vi "Eye Movement Analyser.vi"(7 "Data Output":T12) -> ()   [LabVIEW 2016] (continued)
              frame #1 {
                n995 = local read "Fixed Amplitude"() -> (w2031:bool)
                n996 = case shown="False" w2031 {
                  tunnel: [u8 0 ("Y Scale.Scale Fit") u8 2 ("Y Scale.Scale Fit")] -> w2032
                  frame True {
                  }
                  frame False {
                  }
                }
                n997 = property on="Impulse Trace" class="WFGraph (strict)"("Y Scale.Scale Fit"=w2032) -> ()  [unwired: 2 in, 2 out]
              }
              frame #2 {
                n998 = for {
                  tunnel: w2035 -> [w2041] mode=indexing
                  i -> [w2040]
                  w2036 = 3  # M-STD, M, M+STD
                  n999 = Unbundle By Name(w2041) -> ("Color"=w2038:u32, "Visible"=w2037:bool)
                  n1000 = Multiply(x=w2036, y=w2040) -> (x*y=w2039:i32)
                  n1001 = for {
                    N: w2036 -> [_]
                    tunnel: w2039 -> [w2049]
                    tunnel: w2038 -> [w2042]
                    tunnel: w2037 -> [w2048]
                    i -> [w2046]
                    n1002 = Add(x=w2046, y=w2049) -> (x+y=w2044:i32)
                    n1003 = Equal?(x=w2046, y=1) -> (x = y?=w2047:bool)
                    n1004 = case shown="True" w2047 {
                      tunnel: [u8 0 ("Plot.Line Width") u8 5 ("Plot.Line Width")] -> w2043
                      frame False {
                      }
                      frame True {
                      }
                    }
                    n1005 = property on="Impulse Trace" class="WFGraph (strict)"("Active Plot"=w2044, "Plot.Plot Color"=w2042, "Plot.Visible"=w2048, "Plot.Line Width"=w2043, "Plot.Fill/Pt. Color"=w2042) -> ()  [unwired: 2 in, 2 out]
                  }
                }
              }
            }
          }
          frame Enabled {
          }
        }
      }
      frame "Gain and Phase" {
        n1006 = Bundle By Name(cluster=w2055, "Session saved?"=FALSE) -> (w2054:T17)
        n1007 = local read "Trace"() -> (w2059:i32)
        n1008 = call "Data Analysis.vi"("Data IN"=w2058, "Trace Select"=w2059) -> ("Data OUT"=w2057:T30)  [unwired: 13 in]
      }
      frame "Time Constant Plugin" {
        n1009 = call "Ema to Plugin Data Converter.vi"("Data OUT"=w2064) -> ("Shared Data from EMA"=w2066:T47)  [unwired: 10 in]
        n1010 = Bundle By Name(cluster=w2068, "Session saved?"=FALSE) -> (w2062:T17)
        n1011 = disable-structure shown="Enabled" {
          disable-tunnel: w2066 -> [w2072 w2073]
          disable-tunnel: [w2071 w2073] -> w2065
          frame Disabled {
            n1012 = call "Time Constant - Plugin Main.vi"("Shared Data from EMA"=w2072) -> ("Shared Data to EMA"=w2071:T48)  [unwired: 10 in]
          }
          frame Enabled {
          }
        }
        n1013 = call "Plugin to Ema Data Converter.vi"("Shared Data from EMA in"=w2065, "Data OUT in"=w2064) -> ("Data OUT out"=w2063:T30)  [unwired: 9 in]
      }
      frame "Desaccade Time Data" {
        w2074 = T14[] [enum."Generate New Time Plot", enum."Generate New Impulse Plot"] items=["--- System ---", "Panel Monitoring", "Check Save Status", "Initialize", "Initialise GUI", "Quit", "--- Import ---", "Desaccade Time Data", "Desaccade Time Data Background", "Paint Delete", "Load Batch Log File", "Make Batch List", "Update Batch List", "Delete Batch List", "Delete Temporary LVS", "Save Temporary LVS", "Check for Batch LVS", "Process 3D Chinchilla", "Find default parameter", "Mars3D old", "Chair", "EyeSeeCam", "Open last session", "Save RAW", "Auto Impulse Parameter", "Save Image", "Wireless", "Process Coils Data", "Process JHOC Data", "Process Animal Data", "Australian Data", "ASCII", "Mars 3D", "Mars 3D Training", "Position Mean Plugin", "plot generator plugin", "Human VOG system", "Optotrak", "spline", "COR", "galvanic", "Generate New Time Plot", "Make off and gains permanent", "Generate New Impulse Plot", "Defer Impulse Plot", "Fill Impulse Plot Data", "Scale Impulse Plot", "Un-Defer Impulse Plot", "Snap Impulse Cursor", "Extract Saccades", "Impulse Analyser", "NTA", "Acceleration", "Saccade Velocity", "Horizontal Align", "Vertical Align", "Delete Impulse", "Cut Before", "Cut After", "Filter Data", "Undo Last", "Redo", "Mean and STD", "Group Analyser", "Generate Report", "Phase Plots", "Gain and Phase", "Example Plugin", "Time Constant Plugin", "Export Data", "Export Time Series Data", "Append Data", "Save Data", "Load Data", "Cut in Range", "Keep in range", "Stop"] ("State stack IN")
        n1014 = call "restore Datafile from Backup.vi"("Data OUT in"=w2077, "Statemachine Data OUT"=w2076) -> ("Data OUT out"=w2075:T30)  [unwired: 9 in]
        n1015 = call "Ema to Plugin Data Converter.vi"("Data OUT"=w2075) -> ("Shared Data from EMA"=w2082:T47)  [unwired: 10 in]
        n1016 = Bundle By Name(cluster=w2084, "Session saved?"=FALSE) -> (w2079:T17)
        n1017 = call "Plugin Main - Desaccade time data.vi"("Background Mode"=FALSE, "Shared Data from EMA"=w2082) -> ("Shared Data from EMA 2"=w2081:T47)  [unwired: 9 in]
        n1018 = call "Plugin to Ema Data Converter.vi"("Shared Data from EMA in"=w2081, "Data OUT in"=w2077) -> ("Data OUT out"=w2080:T30)  [unwired: 9 in]
      }
      frame "Desaccade Time Data Background" {
        n1019 = call "restore Datafile from Backup.vi"("Data OUT in"=w2087, "Statemachine Data OUT"=w2088) -> ("Data OUT out"=w2086:T30)  [unwired: 9 in]
        n1020 = call "Ema to Plugin Data Converter.vi"("Data OUT"=w2086) -> ("Shared Data from EMA"=w2093:T47)  [unwired: 10 in]
        n1021 = Bundle By Name(cluster=w2095, "Session saved?"=FALSE) -> (w2090:T17)
        n1022 = call "Plugin Main - Desaccade time data.vi"("Background Mode"=TRUE, "Shared Data from EMA"=w2093) -> ("Shared Data from EMA 2"=w2092:T47)  [unwired: 9 in]
        n1023 = call "Plugin to Ema Data Converter.vi"("Shared Data from EMA in"=w2092, "Data OUT in"=w2086) -> ("Data OUT out"=w2091:T30)  [unwired: 9 in]
      }
      frame "Phase Plots" {
        n1024 = Unbundle By Name(w2104) -> ("desacc"=w2100:T31, "Impulse Positions"=w2103:T11)
        n1025 = local read "Data Output"() -> (w2102:T12)
        n1026 = call "Phase Plots.vi"("Impulse Positions"=w2103, "Data Output"=w2102, "desacc"=w2100) -> ()  [unwired: 5 in]
      }
      frame "Generate Report" {
        n1027 = call "Generate Report.vi"("Data In"=w2106) -> ()  [unwired: 9 in]
      }
      frame "NTA" {
        w2137 = u16 5 items=["Hx Position-in-Head", "Hy Position-in-Head", "Hz Position-in-Head", "Hx Velocity-in-Head", "Hy Velocity-in-Head", "Hz Velocity-in-Head", "Hl Velocity-in-Head", "Hr Velocity-in-Head", "Lx Position-in-Head", "Ly Position-in-Head", "Lz Position-in-Head", "Lx Velocity-in-Head", "Ly Velocity-in-Head", "Lz Velocity-in-Head", "Ll Velocity-in-Head", "Lr Velocity-in-Head", "Rx Position-in-Head", "Ry Position-in-Head", "Rz Position-in-Head", "Rx Velocity-in-Head", "Ry Velocity-in-Head", "Rz Velocity-in-Head", "Rl Velocity-in-Head", "Rr Velocity-in-Head", "Button", "Ascension X", "Ascension X Vel", "Ascension Y", "Ascension Y Vel", "Ascension Z", "Ascension Z Vel", " "] ("List 2")
        w2136 = u16 4 items=["Hx Position-in-Head", "Hy Position-in-Head", "Hz Position-in-Head", "Hx Velocity-in-Head", "Hy Velocity-in-Head", "Hz Velocity-in-Head", "Hl Velocity-in-Head", "Hr Velocity-in-Head", "Lx Position-in-Head", "Ly Position-in-Head", "Lz Position-in-Head", "Lx Velocity-in-Head", "Ly Velocity-in-Head", "Lz Velocity-in-Head", "Ll Velocity-in-Head", "Lr Velocity-in-Head", "Rx Position-in-Head", "Ry Position-in-Head", "Rz Position-in-Head", "Rx Velocity-in-Head", "Ry Velocity-in-Head", "Rz Velocity-in-Head", "Rl Velocity-in-Head", "Rr Velocity-in-Head", "Button", "Ascension X", "Ascension X Vel", "Ascension Y", "Ascension Y Vel", "Ascension Z", "Ascension Z Vel", " "] ("List 2")
        w2135 = u16 3 items=["Hx Position-in-Head", "Hy Position-in-Head", "Hz Position-in-Head", "Hx Velocity-in-Head", "Hy Velocity-in-Head", "Hz Velocity-in-Head", "Hl Velocity-in-Head", "Hr Velocity-in-Head", "Lx Position-in-Head", "Ly Position-in-Head", "Lz Position-in-Head", "Lx Velocity-in-Head", "Ly Velocity-in-Head", "Lz Velocity-in-Head", "Ll Velocity-in-Head", "Lr Velocity-in-Head", "Rx Position-in-Head", "Ry Position-in-Head", "Rz Position-in-Head", "Rx Velocity-in-Head", "Ry Velocity-in-Head", "Rz Velocity-in-Head", "Rl Velocity-in-Head", "Rr Velocity-in-Head", "Button", "Ascension X", "Ascension X Vel", "Ascension Y", "Ascension Y Vel", "Ascension Z", "Ascension Z Vel", " "] ("List 2")
        w2149 = u16 21 items=["Hx Position-in-Head", "Hy Position-in-Head", "Hz Position-in-Head", "Hx Velocity-in-Head", "Hy Velocity-in-Head", "Hz Velocity-in-Head", "Hl Velocity-in-Head", "Hr Velocity-in-Head", "Lx Position-in-Head", "Ly Position-in-Head", "Lz Position-in-Head", "Lx Velocity-in-Head", "Ly Velocity-in-Head", "Lz Velocity-in-Head", "Ll Velocity-in-Head", "Lr Velocity-in-Head", "Rx Position-in-Head", "Ry Position-in-Head", "Rz Position-in-Head", "Rx Velocity-in-Head", "Ry Velocity-in-Head", "Rz Velocity-in-Head", "Rl Velocity-in-Head", "Rr Velocity-in-Head", "Button", "Ascension X", "Ascension X Vel", "Ascension Y", "Ascension Y Vel", "Ascension Z", "Ascension Z Vel", " "] ("List 2")
        w2150 = u16 20 items=["Hx Position-in-Head", "Hy Position-in-Head", "Hz Position-in-Head", "Hx Velocity-in-Head", "Hy Velocity-in-Head", "Hz Velocity-in-Head", "Hl Velocity-in-Head", "Hr Velocity-in-Head", "Lx Position-in-Head", "Ly Position-in-Head", "Lz Position-in-Head", "Lx Velocity-in-Head", "Ly Velocity-in-Head", "Lz Velocity-in-Head", "Ll Velocity-in-Head", "Lr Velocity-in-Head", "Rx Position-in-Head", "Ry Position-in-Head", "Rz Position-in-Head", "Rx Velocity-in-Head", "Ry Velocity-in-Head", "Rz Velocity-in-Head", "Rl Velocity-in-Head", "Rr Velocity-in-Head", "Button", "Ascension X", "Ascension X Vel", "Ascension Y", "Ascension Y Vel", "Ascension Z", "Ascension Z Vel", " "] ("List 2")
        w2151 = u16 19 items=["Hx Position-in-Head", "Hy Position-in-Head", "Hz Position-in-Head", "Hx Velocity-in-Head", "Hy Velocity-in-Head", "Hz Velocity-in-Head", "Hl Velocity-in-Head", "Hr Velocity-in-Head", "Lx Position-in-Head", "Ly Position-in-Head", "Lz Position-in-Head", "Lx Velocity-in-Head", "Ly Velocity-in-Head", "Lz Velocity-in-Head", "Ll Velocity-in-Head", "Lr Velocity-in-Head", "Rx Position-in-Head", "Ry Position-in-Head", "Rz Position-in-Head", "Rx Velocity-in-Head", "Ry Velocity-in-Head", "Rz Velocity-in-Head", "Rl Velocity-in-Head", "Rr Velocity-in-Head", "Button", "Ascension X", "Ascension X Vel", "Ascension Y", "Ascension Y Vel", "Ascension Z", "Ascension Z Vel", " "] ("List 2")
        w2154 = u16 13 items=["Hx Position-in-Head", "Hy Position-in-Head", "Hz Position-in-Head", "Hx Velocity-in-Head", "Hy Velocity-in-Head", "Hz Velocity-in-Head", "Hl Velocity-in-Head", "Hr Velocity-in-Head", "Lx Position-in-Head", "Ly Position-in-Head", "Lz Position-in-Head", "Lx Velocity-in-Head", "Ly Velocity-in-Head", "Lz Velocity-in-Head", "Ll Velocity-in-Head", "Lr Velocity-in-Head", "Rx Position-in-Head", "Ry Position-in-Head", "Rz Position-in-Head", "Rx Velocity-in-Head", "Ry Velocity-in-Head", "Rz Velocity-in-Head", "Rl Velocity-in-Head", "Rr Velocity-in-Head", "Button", "Ascension X", "Ascension X Vel", "Ascension Y", "Ascension Y Vel", "Ascension Z", "Ascension Z Vel", " "] ("List 2")
        w2153 = u16 12 items=["Hx Position-in-Head", "Hy Position-in-Head", "Hz Position-in-Head", "Hx Velocity-in-Head", "Hy Velocity-in-Head", "Hz Velocity-in-Head", "Hl Velocity-in-Head", "Hr Velocity-in-Head", "Lx Position-in-Head", "Ly Position-in-Head", "Lz Position-in-Head", "Lx Velocity-in-Head", "Ly Velocity-in-Head", "Lz Velocity-in-Head", "Ll Velocity-in-Head", "Lr Velocity-in-Head", "Rx Position-in-Head", "Ry Position-in-Head", "Rz Position-in-Head", "Rx Velocity-in-Head", "Ry Velocity-in-Head", "Rz Velocity-in-Head", "Rl Velocity-in-Head", "Rr Velocity-in-Head", "Button", "Ascension X", "Ascension X Vel", "Ascension Y", "Ascension Y Vel", "Ascension Z", "Ascension Z Vel", " "] ("List 2")
        w2152 = u16 11 items=["Hx Position-in-Head", "Hy Position-in-Head", "Hz Position-in-Head", "Hx Velocity-in-Head", "Hy Velocity-in-Head", "Hz Velocity-in-Head", "Hl Velocity-in-Head", "Hr Velocity-in-Head", "Lx Position-in-Head", "Ly Position-in-Head", "Lz Position-in-Head", "Lx Velocity-in-Head", "Ly Velocity-in-Head", "Lz Velocity-in-Head", "Ll Velocity-in-Head", "Lr Velocity-in-Head", "Rx Position-in-Head", "Ry Position-in-Head", "Rz Position-in-Head", "Rx Velocity-in-Head", "Ry Velocity-in-Head", "Rz Velocity-in-Head", "Rl Velocity-in-Head", "Rr Velocity-in-Head", "Button", "Ascension X", "Ascension X Vel", "Ascension Y", "Ascension Y Vel", "Ascension Z", "Ascension Z Vel", " "] ("List 2")
        n1028 = Unbundle By Name(w2114) -> ("Impulse Positions"=w2156:T11)
        n1029 = local read "Data Output"() -> (w2117:T12)
        n1030 = Unbundle By Name(w2117) -> ("Data Channels"=w2130:dbl[][], "Channel List"=w2125:string[])
        n1031 = Array Size(array=w2125) -> (size(s)=w2127:i32)
        n1032 = Decrement(x=w2127) -> (x-1=w2126:i32)
        n1033 = Array Subset(array=w2125, index=0, length=w2126) -> ()  [unwired: 1 out]
        n1034 = Build Array (concatenate)(w2125, string[] ["Lx Velocity-in-Eye", "Ly Velocity-in-Eye", "Lz Velocity-in-Eye", "Rx Velocity-in-Eye", "Ry Velocity-in-Eye", "Rz Velocity-in-Eye", "Hx Velocity-in-Left Eye", "Hy Velocity-in-Left Eye", "Hz Velocity-in-Left Eye", "Hx Velocity-in-Right-Eye", "Hy Velocity-in-Right-Eye", "Hz Velocity-in-Right-Eye"]) -> (w2115:string[])
        n1035 = Index Array(array=w2130, index (row)=w2135) -> (element=w2138:dbl[])  [unwired: 1 in]
        n1036 = Index Array(array=w2130, index (row)=w2136) -> (element=w2139:dbl[])  [unwired: 1 in]
        n1037 = Index Array(array=w2130, index (row)=w2137) -> (element=w2140:dbl[])  [unwired: 1 in]
        n1038 = case shown="\"Near Left 20\"" "Target position" {
          tunnel: [w2158 w2159 w2161 w2163 w2165 w2166 w2167 w2168] -> w2120
          tunnel: [w2158 w2159 w2160 w2162 w2164 w2166 w2167 w2168] -> w2121
          frame "Far Left 20", Default {
            w2158 = -20.0 ("Angle")
          }
          frame "Far Left 30" {
            w2159 = -30.0 ("Angle")
          }
          frame "Near 0" {
            w2160 = 12.0  # Left
            w2161 = -12.0  # Right
          }
          frame "Near Left 20" {
            w2162 = -8.0  # Left
            w2163 = -29.0  # Right
          }
          frame "Near Right 20" {
            w2164 = 29.0  # Left
            w2165 = 8.0  # Right
          }
          frame "Far 0" {
            w2166 = 0.0 ("Angle")
          }
          frame "Far Right 20" {
            w2167 = 20.0 ("Angle")
          }
          frame "Far right 30" {
            w2168 = 30.0 ("Angle")
          }
        }
        n1039 = Index Array(array=w2130, index (row)=w2152) -> (element=w2148:dbl[])  [unwired: 1 in]
        n1040 = Index Array(array=w2130, index (row)=w2153) -> (element=w2146:dbl[])  [unwired: 1 in]
        n1041 = Index Array(array=w2130, index (row)=w2154) -> (element=w2144:dbl[])  [unwired: 1 in]
        n1042 = Index Array(array=w2130, index (row)=w2151) -> (element=w2147:dbl[])  [unwired: 1 in]
        n1043 = Index Array(array=w2130, index (row)=w2150) -> (element=w2145:dbl[])  [unwired: 1 in]
        n1044 = Index Array(array=w2130, index (row)=w2149) -> (element=w2143:dbl[])  [unwired: 1 in]
        n1045 = Build Array(w2138, w2139, w2140) -> (w2118:dbl[][])
        n1046 = Build Array(w2148, w2146, w2144) -> (w2133:dbl[][])
        n1047 = Build Array(w2147, w2145, w2143) -> (w2134:dbl[][])
        n1048 = call "Change coord.vi"("Principal Planes"=w2118, "Angle"=w2121) -> ("New Planes"=w2123:dbl[][])
        n1049 = call "Change coord.vi"("Principal Planes"=w2118, "Angle"=w2120) -> ("New Planes"=w2122:dbl[][])
        n1050 = call "Change coord.vi"("Principal Planes"=w2133, "Angle"=w2121) -> ("New Planes"=w2131:dbl[][])
        n1051 = call "Change coord.vi"("Principal Planes"=w2134, "Angle"=w2120) -> ("New Planes"=w2132:dbl[][])
        n1052 = Unbundle By Name(w2114) -> ("Impulse Positions"=w2141:T11, "No. Imp"=w2142:i32)
        n1053 = Build Array (concatenate)(w2130, w2131, w2132, w2123, w2122) -> (w2129:dbl[][])
        n1054 = Bundle By Name(cluster=w2117, "Data Channels"=w2129, "Channel List"=w2115) -> (w2116:T12)
        n1055 = local write "Data Output"(w2116) -> ()
        n1056 = local write "Impulse Positions"(w2141) -> ()
        n1057 = local write "No. Imp"(w2142) -> ()
        n1058 = case shown="True" "Head coord" {
          tunnel: w2156 -> [w2170 w2172]
          tunnel: w2116 -> [w2169 w2171]
          frame False {
            n1059 = call "Generate Report work with Zee 2.vi"("Impulse Positions"=w2170, "Impulse Data"=w2169) -> ()  [unwired: 8 in]
          }
          frame True {
            n1060 = call "Generate Report work with Zee.vi"("Impulse Positions"=w2172, "Impulse Data"=w2171) -> ()  [unwired: 8 in]
          }
        }
      }
      frame "Acceleration" {
        w2204 = u16 5 items=["Hx Position-in-Head", "Hy Position-in-Head", "Hz Position-in-Head", "Hx Velocity-in-Head", "Hy Velocity-in-Head", "Hz Velocity-in-Head", "Hl Velocity-in-Head", "Hr Velocity-in-Head", "Lx Position-in-Head", "Ly Position-in-Head", "Lz Position-in-Head", "Lx Velocity-in-Head", "Ly Velocity-in-Head", "Lz Velocity-in-Head", "Ll Velocity-in-Head", "Lr Velocity-in-Head", "Rx Position-in-Head", "Ry Position-in-Head", "Rz Position-in-Head", "Rx Velocity-in-Head", "Ry Velocity-in-Head", "Rz Velocity-in-Head", "Rl Velocity-in-Head", "Rr Velocity-in-Head", "Button", "Ascension X", "Ascension X Vel", "Ascension Y", "Ascension Y Vel", "Ascension Z", "Ascension Z Vel", " "] ("List 2")
        w2203 = u16 4 items=["Hx Position-in-Head", "Hy Position-in-Head", "Hz Position-in-Head", "Hx Velocity-in-Head", "Hy Velocity-in-Head", "Hz Velocity-in-Head", "Hl Velocity-in-Head", "Hr Velocity-in-Head", "Lx Position-in-Head", "Ly Position-in-Head", "Lz Position-in-Head", "Lx Velocity-in-Head", "Ly Velocity-in-Head", "Lz Velocity-in-Head", "Ll Velocity-in-Head", "Lr Velocity-in-Head", "Rx Position-in-Head", "Ry Position-in-Head", "Rz Position-in-Head", "Rx Velocity-in-Head", "Ry Velocity-in-Head", "Rz Velocity-in-Head", "Rl Velocity-in-Head", "Rr Velocity-in-Head", "Button", "Ascension X", "Ascension X Vel", "Ascension Y", "Ascension Y Vel", "Ascension Z", "Ascension Z Vel", " "] ("List 2")
        w2202 = u16 3 items=["Hx Position-in-Head", "Hy Position-in-Head", "Hz Position-in-Head", "Hx Velocity-in-Head", "Hy Velocity-in-Head", "Hz Velocity-in-Head", "Hl Velocity-in-Head", "Hr Velocity-in-Head", "Lx Position-in-Head", "Ly Position-in-Head", "Lz Position-in-Head", "Lx Velocity-in-Head", "Ly Velocity-in-Head", "Lz Velocity-in-Head", "Ll Velocity-in-Head", "Lr Velocity-in-Head", "Rx Position-in-Head", "Ry Position-in-Head", "Rz Position-in-Head", "Rx Velocity-in-Head", "Ry Velocity-in-Head", "Rz Velocity-in-Head", "Rl Velocity-in-Head", "Rr Velocity-in-Head", "Button", "Ascension X", "Ascension X Vel", "Ascension Y", "Ascension Y Vel", "Ascension Z", "Ascension Z Vel", " "] ("List 2")
        w2205 = u16 21 items=["Hx Position-in-Head", "Hy Position-in-Head", "Hz Position-in-Head", "Hx Velocity-in-Head", "Hy Velocity-in-Head", "Hz Velocity-in-Head", "Hl Velocity-in-Head", "Hr Velocity-in-Head", "Lx Position-in-Head", "Ly Position-in-Head", "Lz Position-in-Head", "Lx Velocity-in-Head", "Ly Velocity-in-Head", "Lz Velocity-in-Head", "Ll Velocity-in-Head", "Lr Velocity-in-Head", "Rx Position-in-Head", "Ry Position-in-Head", "Rz Position-in-Head", "Rx Velocity-in-Head", "Ry Velocity-in-Head", "Rz Velocity-in-Head", "Rl Velocity-in-Head", "Rr Velocity-in-Head", "Button", "Ascension X", "Ascension X Vel", "Ascension Y", "Ascension Y Vel", "Ascension Z", "Ascension Z Vel", " "] ("List 2")
        w2206 = u16 20 items=["Hx Position-in-Head", "Hy Position-in-Head", "Hz Position-in-Head", "Hx Velocity-in-Head", "Hy Velocity-in-Head", "Hz Velocity-in-Head", "Hl Velocity-in-Head", "Hr Velocity-in-Head", "Lx Position-in-Head", "Ly Position-in-Head", "Lz Position-in-Head", "Lx Velocity-in-Head", "Ly Velocity-in-Head", "Lz Velocity-in-Head", "Ll Velocity-in-Head", "Lr Velocity-in-Head", "Rx Position-in-Head", "Ry Position-in-Head", "Rz Position-in-Head", "Rx Velocity-in-Head", "Ry Velocity-in-Head", "Rz Velocity-in-Head", "Rl Velocity-in-Head", "Rr Velocity-in-Head", "Button", "Ascension X", "Ascension X Vel", "Ascension Y", "Ascension Y Vel", "Ascension Z", "Ascension Z Vel", " "] ("List 2")
        w2207 = u16 19 items=["Hx Position-in-Head", "Hy Position-in-Head", "Hz Position-in-Head", "Hx Velocity-in-Head", "Hy Velocity-in-Head", "Hz Velocity-in-Head", "Hl Velocity-in-Head", "Hr Velocity-in-Head", "Lx Position-in-Head", "Ly Position-in-Head", "Lz Position-in-Head", "Lx Velocity-in-Head", "Ly Velocity-in-Head", "Lz Velocity-in-Head", "Ll Velocity-in-Head", "Lr Velocity-in-Head", "Rx Position-in-Head", "Ry Position-in-Head", "Rz Position-in-Head", "Rx Velocity-in-Head", "Ry Velocity-in-Head", "Rz Velocity-in-Head", "Rl Velocity-in-Head", "Rr Velocity-in-Head", "Button", "Ascension X", "Ascension X Vel", "Ascension Y", "Ascension Y Vel", "Ascension Z", "Ascension Z Vel", " "] ("List 2")
        w2210 = u16 13 items=["Hx Position-in-Head", "Hy Position-in-Head", "Hz Position-in-Head", "Hx Velocity-in-Head", "Hy Velocity-in-Head", "Hz Velocity-in-Head", "Hl Velocity-in-Head", "Hr Velocity-in-Head", "Lx Position-in-Head", "Ly Position-in-Head", "Lz Position-in-Head", "Lx Velocity-in-Head", "Ly Velocity-in-Head", "Lz Velocity-in-Head", "Ll Velocity-in-Head", "Lr Velocity-in-Head", "Rx Position-in-Head", "Ry Position-in-Head", "Rz Position-in-Head", "Rx Velocity-in-Head", "Ry Velocity-in-Head", "Rz Velocity-in-Head", "Rl Velocity-in-Head", "Rr Velocity-in-Head", "Button", "Ascension X", "Ascension X Vel", "Ascension Y", "Ascension Y Vel", "Ascension Z", "Ascension Z Vel", " "] ("List 2")
        w2209 = u16 12 items=["Hx Position-in-Head", "Hy Position-in-Head", "Hz Position-in-Head", "Hx Velocity-in-Head", "Hy Velocity-in-Head", "Hz Velocity-in-Head", "Hl Velocity-in-Head", "Hr Velocity-in-Head", "Lx Position-in-Head", "Ly Position-in-Head", "Lz Position-in-Head", "Lx Velocity-in-Head", "Ly Velocity-in-Head", "Lz Velocity-in-Head", "Ll Velocity-in-Head", "Lr Velocity-in-Head", "Rx Position-in-Head", "Ry Position-in-Head", "Rz Position-in-Head", "Rx Velocity-in-Head", "Ry Velocity-in-Head", "Rz Velocity-in-Head", "Rl Velocity-in-Head", "Rr Velocity-in-Head", "Button", "Ascension X", "Ascension X Vel", "Ascension Y", "Ascension Y Vel", "Ascension Z", "Ascension Z Vel", " "] ("List 2")
        w2208 = u16 11 items=["Hx Position-in-Head", "Hy Position-in-Head", "Hz Position-in-Head", "Hx Velocity-in-Head", "Hy Velocity-in-Head", "Hz Velocity-in-Head", "Hl Velocity-in-Head", "Hr Velocity-in-Head", "Lx Position-in-Head", "Ly Position-in-Head", "Lz Position-in-Head", "Lx Velocity-in-Head", "Ly Velocity-in-Head", "Lz Velocity-in-Head", "Ll Velocity-in-Head", "Lr Velocity-in-Head", "Rx Position-in-Head", "Ry Position-in-Head", "Rz Position-in-Head", "Rx Velocity-in-Head", "Ry Velocity-in-Head", "Rz Velocity-in-Head", "Rl Velocity-in-Head", "Rr Velocity-in-Head", "Button", "Ascension X", "Ascension X Vel", "Ascension Y", "Ascension Y Vel", "Ascension Z", "Ascension Z Vel", " "] ("List 2")
        n1061 = Unbundle By Name(w2174) -> ("Data File.Data Channels"=w2201:dbl[][], "Data File.Channel List"=w2186:string[], "Data File.Sample Rate"=w2189:i32)
        n1062 = Array Size(array=w2186) -> (size(s)=w2185:i32)
        n1063 = Decrement(x=w2185) -> (x-1=w2180:i32)
        n1064 = Array Subset(array=w2186, index=0, length=w2180) -> (w2184:string[])
        n1065 = Build Array (concatenate)(w2184, string[] ["Lx Acc-in-Head", "Ly Acc-in-Head", "Lz Acc-in-Head", "Rx Acc-in-Head", "Ry Acc-in-Head", "Rz Acc-in-Head", "Hx Acc-in-Head", "Hy Acc-in-Head", "Hz Acc-in-Head", ""]) -> (w2211:string[])
        n1066 = Index Array(array=w2201, index (row)=w2202) -> (element=w2193:dbl[])  [unwired: 1 in]
        n1067 = Index Array(array=w2201, index (row)=w2203) -> (element=w2192:dbl[])  [unwired: 1 in]
        n1068 = Index Array(array=w2201, index (row)=w2204) -> (element=w2191:dbl[])  [unwired: 1 in]
        n1069 = Index Array(array=w2201, index (row)=w2208) -> (element=w2199:dbl[])  [unwired: 1 in]
        n1070 = Index Array(array=w2201, index (row)=w2209) -> (element=w2198:dbl[])  [unwired: 1 in]
        n1071 = Index Array(array=w2201, index (row)=w2210) -> (element=w2197:dbl[])  [unwired: 1 in]
        n1072 = Index Array(array=w2201, index (row)=w2207) -> (element=w2196:dbl[])  [unwired: 1 in]
        n1073 = Index Array(array=w2201, index (row)=w2206) -> (element=w2195:dbl[])  [unwired: 1 in]
        n1074 = Index Array(array=w2201, index (row)=w2205) -> (element=w2194:dbl[])  [unwired: 1 in]
        n1075 = Build Array(w2199, w2198, w2197, w2196, w2195, w2194, w2193, w2192, w2191) -> (w2190:dbl[][])
        n1076 = call "Differentiate 3D.vi"("Sample Rate 4"=w2189, "Data (in)"=w2190) -> ("Data (differentiated)"=w2188:dbl[][])  [unwired: 3 in]
        n1077 = Array Subset(array=w2201, index (row)=0 ("index"), length (row)=w2180) -> (w2182:dbl[][])  [unwired: 2 in]
        n1078 = Unbundle By Name(w2179) -> ("Impulse Positions"=w2178:T11, "No. Imp"=w2177:i32)
        n1079 = Build Array (concatenate)(w2182, w2188) -> (w2200:dbl[][])
        n1080 = Bundle By Name(cluster=w2174, "Data File.Data Channels"=w2200, "Data File.Channel List"=w2211) -> (w2173:T30)
        n1081 = local write "Impulse Positions"(w2178) -> ()
        n1082 = local write "No. Imp"(w2177) -> ()
      }
      frame "Group Analyser" {
        n1083 = call "Group Analyser.vi"() -> ()  [unwired: 8 in]
      }
      frame "Check Save Status" {
        n1084 = Unbundle By Name(w2222) -> ("Session saved?"=w2224:bool)
        n1085 = case shown="False" w2224 {
          tunnel: [w2231 T22."Center Button" ("Which Button?")] -> w2223
          frame False {
            n1086 = call <vilib>:"Three Button Dialog.vi"("Allow user to close window? (TRUE)"=FALSE, "Window Title (\"\")"="Forgot to save?" ("Window Title (\"\")"), "message"="Current session was not saved!\nDo you want to save now?") -> ("Which Button?"=w2231:T22)  [unwired: 8 in]
          }
          frame True {
          }
        }
        n1087 = case shown="\"Left Button\", Default" w2223 {
          tunnel: [w2228 w2229 w2230] -> w2221
          tunnel: w2220 -> [w2226 w2229 _]
          frame "Left Button", Default {
            w2227 = T14[] [enum."Save Data"] items=["--- System ---", "Panel Monitoring", "Check Save Status", "Initialize", "Initialise GUI", "Quit", "--- Import ---", "Desaccade Time Data", "Desaccade Time Data Background", "Paint Delete", "Load Batch Log File", "Make Batch List", "Update Batch List", "Delete Batch List", "Delete Temporary LVS", "Save Temporary LVS", "Check for Batch LVS", "Process 3D Chinchilla", "Find default parameter", "Mars3D old", "Chair", "EyeSeeCam", "Open last session", "Save RAW", "Auto Impulse Parameter", "Save Image", "Wireless", "Process Coils Data", "Process JHOC Data", "Process Animal Data", "Australian Data", "ASCII", "Mars 3D", "Mars 3D Training", "Position Mean Plugin", "plot generator plugin", "Human VOG system", "Optotrak", "spline", "COR", "galvanic", "Generate New Time Plot", "Make off and gains permanent", "Generate New Impulse Plot", "Defer Impulse Plot", "Fill Impulse Plot Data", "Scale Impulse Plot", "Un-Defer Impulse Plot", "Snap Impulse Cursor", "Extract Saccades", "Impulse Analyser", "NTA", "Acceleration", "Saccade Velocity", "Horizontal Align", "Vertical Align", "Delete Impulse", "Cut Before", "Cut After", "Filter Data", "Undo Last", "Redo", "Mean and STD", "Group Analyser", "Generate Report", "Phase Plots", "Gain and Phase", "Example Plugin", "Time Constant Plugin", "Export Data", "Export Time Series Data", "Append Data", "Save Data", "Load Data", "Cut in Range", "Keep in range", "Stop"] ("State Stack (out)")
            n1088 = Build Array (concatenate)(w2227, w2226) -> (w2228:T14[])
          }
          frame "Center Button" {
          }
          frame "Right Button" {
            w2230 = T14[] [enum."Panel Monitoring"] items=["--- System ---", "Panel Monitoring", "Check Save Status", "Initialize", "Initialise GUI", "Quit", "--- Import ---", "Desaccade Time Data", "Desaccade Time Data Background", "Paint Delete", "Load Batch Log File", "Make Batch List", "Update Batch List", "Delete Batch List", "Delete Temporary LVS", "Save Temporary LVS", "Check for Batch LVS", "Process 3D Chinchilla", "Find default parameter", "Mars3D old", "Chair", "EyeSeeCam", "Open last session", "Save RAW", "Auto Impulse Parameter", "Save Image", "Wireless", "Process Coils Data", "Process JHOC Data", "Process Animal Data", "Australian Data", "ASCII", "Mars 3D", "Mars 3D Training", "Position Mean Plugin", "plot generator plugin", "Human VOG system", "Optotrak", "spline", "COR", "galvanic", "Generate New Time Plot", "Make off and gains permanent", "Generate New Impulse Plot", "Defer Impulse Plot", "Fill Impulse Plot Data", "Scale Impulse Plot", "Un-Defer Impulse Plot", "Snap Impulse Cursor", "Extract Saccades", "Impulse Analyser", "NTA", "Acceleration", "Saccade Velocity", "Horizontal Align", "Vertical Align", "Delete Impulse", "Cut Before", "Cut After", "Filter Data", "Undo Last", "Redo", "Mean and STD", "Group Analyser", "Generate Report", "Phase Plots", "Gain and Phase", "Example Plugin", "Time Constant Plugin", "Export Data", "Export Time Series Data", "Append Data", "Save Data", "Load Data", "Cut in Range", "Keep in range", "Stop"] ("State Stack (out)")
          }
        }
      }
      frame "Save Data" {
        # "Get path to save at. Use the experiment data path if a valid path is not specified."
        # "Get data"
        # "Open file dialog so the user can specify a file to save the data into."
        # "delete extention"
        n1089 = local read "filename"() -> (w2250:string)
        n1090 = local read "Data Output"() -> (w2261:T12)
        n1091 = Unbundle By Name(w2238) -> ("EMA Version"=w2243:string)
        n1092 = local read "LVS data path"() -> (w2239:path)
        n1093 = Unbundle By Name(w2238) -> ("Experiment data path"=w2237:path)
        n1094 = String Length(string=w2250) -> (length=w2253:i32)
        n1095 = Subtract(x=w2253, y=4) -> (x-y=w2252:i32)
        n1096 = Bundle("Data Output"=w2261, "Data OUT"=w2238) -> (w2262:T39)  [unwired: 1 in]
        n1097 = call-poly <userlib>:"File Exists__ogtk.vi"("file path"=w2239) -> ("is directory"=w2242:bool, "exists"=w2241:bool)  [unwired: 6 in]
        n1098 = String Subset(string=w2250, length (rest)=w2252) -> (substring=w2249:string)  [unwired: 1 in]
        n1099 = And(x=w2242, y=w2241) -> (x .and. y?=w2240:bool)
        n1100 = Select(t=w2239, s=w2240, f=w2237) -> (s? t:f=w2236:path)
        n1101 = Search and Replace String(replace all?=TRUE ("replace all? (F)"), input string=w2249, search string=".", replace string="," ("replace string (\"\")")) -> (result string=w2245:string)  [unwired: 4 in, 3 out]
        n1102 = call "File Dialog2"("start path"=w2236, "prompt"="Please Enter Name Of File (NO Postfix):", "default name"=w2245) -> ("selected path"=w2259:path, "cancelled"=w2260:bool)  [unwired: 9 in, 2 out]
        n1103 = case shown="False" w2260 {
          tunnel: w2262 -> [w2274 _]
          tunnel: w2259 -> [w2273 _]
          tunnel: [w2272 FALSE ("T button?")] -> w2257
          tunnel: w2255 -> [w2271 w2304]
          tunnel: [w2268 w2304] -> w2254
          tunnel: w2243 -> [w2266 _]
          frame False {
            # "Dialog not cancelled. Save the data."
            n1104 = disable-structure shown="Enabled" {
              disable-tunnel: w2274 -> [w2291 w2294]
              disable-tunnel: w2273 -> [w2290 w2293]
              disable-tunnel: w2266 -> [w2277 _]
              frame Disabled {
                # "Flatten data to a string."
                # "Save:\n1. EMA version\n2. Data size\n3. Data"
                # "Add .lvs postfix"
                # "save last path"
                n1105 = Path To String(path=w2290) -> (string=w2283:string)
                n1106 = Strip Path(path=w2290) -> (stripped path=w2275:path)  [unwired: 1 out]
                n1107 = call "File-Suffix.vi"("Substring"=".lvs", "String 2"=w2283) -> ("String"=w2281:string)
                n1108 = local write "LVS data path"(w2275) -> ()
                n1109 = String To Path(string=w2281) -> (path=w2280:path)
                n1110 = Flatten To String(anything=w2291) -> (data string=w2285:string)  [unwired: 3 in, 2 out]
                n1111 = String Length(string=w2285) -> (length=w2287:i32)
                n1112 = call <vilib>:"Open_Create_Replace File.vi"("function (open:0)"=T19."create or replace", "file path"=w2280) -> ("refnum"=w2279:refnum<file>)  [unwired: 6 in, 3 out]
                n1113 = Flatten To String(anything=w2287) -> (data string=w2286:string)  [unwired: 3 in, 2 out]
                n1114 = call <vilib>:"Write File+ (string).vi"("string"=w2277, "refnum"=w2279) -> ("dup refnum"=w2278:refnum<file>)  [unwired: 5 in, 2 out]
                n1115 = call <vilib>:"Write File+ (string).vi"("string"=w2286, "refnum"=w2278) -> ("dup refnum"=w2284:refnum<file>)  [unwired: 5 in, 2 out]
                n1116 = call <vilib>:"Write File+ (string).vi"("string"=w2285, "refnum"=w2284) -> ("dup refnum"=w2289:refnum<file>)  [unwired: 5 in, 2 out]
                n1117 = call <vilib>:"Close File+.vi"("refnum"=w2289) -> ("refnum"=w2276:refnum<file>)  [unwired: 4 in, 2 out]
                n1118 = Close File(refnum=w2276) -> ()  [unwired: 1 in, 2 out]
              }
              frame Enabled {
                n1119 = call "Save LVS.vi"("LVS Data"=w2294, "Path (in)"=w2293) -> ("Path (out)"=w2292:path)  [unwired: 8 in, 1 out]
                n1120 = local write "LVS data path"(w2292) -> ()
              }
            }
            n1121 = Unbundle By Name(w2271) -> ("Save Options"=w2270:bool)
            n1122 = case shown="False" w2270 {
              tunnel: [w2296 w2302] -> w2272
              tunnel: w2271 -> [w2298 w2303]
              tunnel: [w2297 w2303] -> w2269
              frame False {
                # "Save options do not always require an image to be saved. Ask the user if they would like to save an image."
                n1123 = Two Button Dialog(message="Save IMAGE  too?", 1:"No" ("F button name (\"Cancel\")"), 2:"Yes" ("T button name (\"OK\")")) -> (T button?=w2296:bool)
                n1124 = Bundle By Name(cluster=w2298, "Save Options"=TRUE, "Save IMAGE"=w2296) -> (w2297:T17)
              }
              frame True {
                # "Save Options specify to always save an image."
                n1125 = Unbundle By Name(w2303) -> ("Save IMAGE"=w2302:bool)
              }
            }
            n1126 = Bundle By Name(cluster=w2269, "Session saved?"=TRUE) -> (w2268:T17)
          }
          frame True {
            # "Dialog cancelled. Do nothing."
          }
        }
        n1127 = case shown="True" w2257 {
          tunnel: [w2264 w2265] -> w2256
          frame True {
            w2264 = T14[] [enum."Update Batch List", enum."Save Image", enum."Panel Monitoring"] items=["--- System ---", "Panel Monitoring", "Check Save Status", "Initialize", "Initialise GUI", "Quit", "--- Import ---", "Desaccade Time Data", "Desaccade Time Data Background", "Paint Delete", "Load Batch Log File", "Make Batch List", "Update Batch List", "Delete Batch List", "Delete Temporary LVS", "Save Temporary LVS", "Check for Batch LVS", "Process 3D Chinchilla", "Find default parameter", "Mars3D old", "Chair", "EyeSeeCam", "Open last session", "Save RAW", "Auto Impulse Parameter", "Save Image", "Wireless", "Process Coils Data", "Process JHOC Data", "Process Animal Data", "Australian Data", "ASCII", "Mars 3D", "Mars 3D Training", "Position Mean Plugin", "plot generator plugin", "Human VOG system", "Optotrak", "spline", "COR", "galvanic", "Generate New Time Plot", "Make off and gains permanent", "Generate New Impulse Plot", "Defer Impulse Plot", "Fill Impulse Plot Data", "Scale Impulse Plot", "Un-Defer Impulse Plot", "Snap Impulse Cursor", "Extract Saccades", "Impulse Analyser", "NTA", "Acceleration", "Saccade Velocity", "Horizontal Align", "Vertical Align", "Delete Impulse", "Cut Before", "Cut After", "Filter Data", "Undo Last", "Redo", "Mean and STD", "Group Analyser", "Generate Report", "Phase Plots", "Gain and Phase", "Example Plugin", "Time Constant Plugin", "Export Data", "Export Time Series Data", "Append Data", "Save Data", "Load Data", "Cut in Range", "Keep in range", "Stop"] ("State stack IN")
            # "Save images as well before returning to Panel monitoring."
          }
          frame False {
            w2265 = T14[] [enum."Update Batch List", enum."Panel Monitoring"] items=["--- System ---", "Panel Monitoring", "Check Save Status", "Initialize", "Initialise GUI", "Quit", "--- Import ---", "Desaccade Time Data", "Desaccade Time Data Background", "Paint Delete", "Load Batch Log File", "Make Batch List", "Update Batch List", "Delete Batch List", "Delete Temporary LVS", "Save Temporary LVS", "Check for Batch LVS", "Process 3D Chinchilla", "Find default parameter", "Mars3D old", "Chair", "EyeSeeCam", "Open last session", "Save RAW", "Auto Impulse Parameter", "Save Image", "Wireless", "Process Coils Data", "Process JHOC Data", "Process Animal Data", "Australian Data", "ASCII", "Mars 3D", "Mars 3D Training", "Position Mean Plugin", "plot generator plugin", "Human VOG system", "Optotrak", "spline", "COR", "galvanic", "Generate New Time Plot", "Make off and gains permanent", "Generate New Impulse Plot", "Defer Impulse Plot", "Fill Impulse Plot Data", "Scale Impulse Plot", "Un-Defer Impulse Plot", "Snap Impulse Cursor", "Extract Saccades", "Impulse Analyser", "NTA", "Acceleration", "Saccade Velocity", "Horizontal Align", "Vertical Align", "Delete Impulse", "Cut Before", "Cut After", "Filter Data", "Undo Last", "Redo", "Mean and STD", "Group Analyser", "Generate Report", "Phase Plots", "Gain and Phase", "Example Plugin", "Time Constant Plugin", "Export Data", "Export Time Series Data", "Append Data", "Save Data", "Load Data", "Cut in Range", "Keep in range", "Stop"] ("State stack IN")
            # "Don't save any images. Just return to panel monitoring."
          }
        }
      }
      frame "Load Data" {
        n1128 = Unbundle By Name(w2309) -> ("DC file"=w2312:path)
        n1129 = Unbundle By Name(w2311) -> ("Experiment data path"=w2310:path)
        n1130 = Empty String/Path?(string/path=w2312) -> (empty?=w2313:bool)
        n1131 = case shown="True" w2313 {
          tunnel: [w2408 w2411] -> w2315
          tunnel: [FALSE ("cancelled") w2410] -> w2314
          tunnel: w2312 -> [w2408 _]
          tunnel: w2310 -> [_ w2409]
          frame False {
          }
          frame True {
            n1132 = call "File Dialog3"("start path"=w2409, "prompt"="Select Data File:", "pattern (all files)"="*.lvs*" ("pattern")) -> ("selected path"=w2411:path, "cancelled"=w2410:bool)  [unwired: 9 in, 2 out]
          }
        }
        n1133 = disable-structure shown="Enabled" {
          disable-tunnel: w2315 -> [w2323 w2400]
          disable-tunnel: w2314 -> [w2320 w2401]
          disable-tunnel: w2311 -> [w2319 w2399]
          disable-tunnel: [w2318 w2398] -> w2306
          frame Disabled {
            n1134 = case shown="False" w2320 {
              tunnel: w2323 -> [w2328 _]
              tunnel: [w2326 refnum<file> refnum ("dup refnum")] -> w2322
              tunnel: [w2325 "CANCEL" ("string")] -> w2321
              frame False {
                n1135 = call <vilib>:"Open_Create_Replace File.vi"("file path"=w2328) -> ("refnum"=w2327:refnum<file>)  [unwired: 7 in, 3 out]
                n1136 = call <vilib>:"Read File+ (string).vi"("count"=9, "refnum"=w2327) -> ("string"=w2325:string, "dup refnum"=w2326:refnum<file>)  [unwired: 5 in, 3 out]
              }
              frame True {
              }
            }
            n1137 = case shown="\"EMA 2011a\"" w2321 {
              tunnel: w2323 -> [w2357 w2370 w2382 _]
              tunnel: w2319 -> [w2354 w2369 w2386 w2397]
              tunnel: [w2358 w2372 w2388 w2397] -> w2318
              tunnel: w2322 -> [w2356 w2368 w2378 _]
              frame "EMA 2011a" {
                w2363 = 4 ("count")
                # "Keep previous settings"
                n1138 = Strip Path(path=w2357) -> (stripped path=w2332:path, name=w2331:string)
                n1139 = local read "Data Output"() -> (w2361:T12)
                n1140 = local write "loaded filename"(w2357) -> ()
                n1141 = call <vilib>:"Read File+ (string).vi"("count"=w2363, "refnum"=w2356) -> ("string"=w2364:string, "dup refnum"=w2365:refnum<file>)  [unwired: 5 in, 3 out]
                n1142 = Unflatten From String(type=w2363, binary string=w2364) -> (value=w2362:i32)  [unwired: 3 in, 2 out]
                n1143 = Bundle("Data Output"=w2361, "output cluster"=T23 {"Impulse Positions"=[], "Old Impulse positions for Undo"=[], "No. Imp"=0, "Parameter Time Series"=[], "Parameter Impuls Series"=[], "Experiment Parameters"={"Freq"=0.0, "Vel"=0, "Acc"=0, "Stimulus"=""}, "Autosort File"=refnum, "Data File"={"Data Channels"=[], "Sample Rate"=0, "Channel List"=[]}, "Experiment data path"=path "/Macintosh HD/Users/patrick/Studium/Diploma Thesis/Data Analysis", "Image data path"=path "/Macintosh HD/Users/patrick/Studium/Diploma Thesis/Data Analysis", "LVS data path"=path "/Macintosh HD/Users/patrick/Studium/Diploma Thesis/Data Analysis", "Raw copy path"=path "/Macintosh HD/Users/patrick/Studium/Diploma Thesis/Data Analysis", "filename"="No file selected", "desaccading parameters"={"Tolerance"=0, "Acc Range"=0.0, "Sample Rate"=0, "Impulse Plane 2"=enum."Other", "Impulse dir"=FALSE}, "Experiment Parameters 2"={"Subject"="", "Strain"="", "Rotation plane"="", "Experimenter"="", "Trial"=0.0, "Time"=0.0}, "Excel"={"Excel._Application"=refnum, "Use Excel"=FALSE, "Worksheet SINE"=refnum, "Row SINE"=0, "Worksheet TRANS"=refnum, "Row TRANS"=0}, "Session Config File"=refnum, "Autosort Parameter Set"=1, "EMA Version"="", "desacc "={"Threshold 1 [Acc]"=1617.080808080808, "Threshold 2 [% of TH1]"=67, "tolerance"=5, "Search WD "=0.19090909090909092, " always use TH2"=TRUE, "Range"=3.2323232323232323, "Max time"=200.0, "Min time"=20.0}}) -> (w2360:T50)  [unwired: 1 in]
                n1144 = call <vilib>:"Read File+ (string).vi"("count"=w2362, "refnum"=w2365) -> ("string"=w2366:string)  [unwired: 5 in, 4 out]
                n1145 = Unflatten From String(type=w2360, binary string=w2366) -> (value=w2359:T50)  [unwired: 3 in, 2 out]
                n1146 = Unbundle(w2359) -> ("output cluster"=w2353:T23)  [unwired: 1 out]
                n1147 = Unbundle By Name(w2353) -> ("Impulse Positions"=w2352:T11, "No. Imp"=w2351:i32, "Parameter Time Series"=w2350:T2, "Parameter Impuls Series"=w2349:T8, "Experiment Parameters"=w2348:T25, "Autosort File"=w2347:refnum<file>, "Data File"=w2346:T12, "desaccading parameters"=w2345:T37, "Experiment Parameters 2"=w2344:T24, "Session Config File"=w2343:refnum<file>, "Autosort Parameter Set"=w2342:i32, "desacc.Threshold 1 [Acc]"=w2341:dbl, "desacc.Threshold 2 [% of TH1]"=w2340:i32, "desacc.tolerance"=w2339:i32, "desacc.Search WD"=w2338:dbl, "desacc.always use TH2"=w2337:bool, "desacc.Range"=w2336:dbl, "desacc.Max time"=w2335:dbl, "desacc.Min time"=w2334:dbl)  [unwired: 5 out]
                n1148 = Bundle By Name(cluster=w2354, "Impulse Positions"=w2352, "No. Imp"=w2351, "Parameter Time Series"=w2350, "Parameter Impuls Series"=w2349, "Experiment Parameters"=w2348, "Autosort File"=w2347, "Data File"=w2346, "Experiment data path"=w2332, "filename"=w2331, "desaccading parameters"=w2345, "Experiment Parameters 2"=w2344, "Session Config File"=w2343, "Autosort Parameter Set"=w2342, "desacc.Threshold 1 [Acc]"=w2341, "desacc.Threshold 2 [% of TH1]"=w2340, "desacc.tolerance"=w2339, "desacc.Search WD"=w2338, "desacc.always use TH2"=w2337, "desacc.Range"=w2336, "desacc.Max time"=w2335, "desacc.Min time"=w2334, "desacc.Velocity Threshold"=200 ("desacc .Velocity Threshold")) -> (w2358:T30)
              }
              frame "EMA 2011b" {
                n1149 = Strip Path(path=w2370) -> (name=w2371:string)  [unwired: 1 out]
                n1150 = Strip Path(path=w2370) -> (stripped path=w2373:path)  [unwired: 1 out]
                n1151 = local write "loaded filename"(w2370) -> ()
                n1152 = local write "filename"(w2371) -> ()
                n1153 = local write "LVS data path"(w2373) -> ()
                n1154 = call "Load LVS EMA 2010b.vi"("Data OUT in"=w2369, "Byte Stream File in"=w2368) -> ("Byte Stream File out"=w2367:refnum<file>, "Data OUT out"=w2372:T30)  [unwired: 8 in]
                n1155 = Close File(refnum=w2367) -> ()  [unwired: 1 in, 2 out]
              }
              frame "????", Default {
                w2393 = 4 ("count")
                # "Old EMA Versions"
                n1156 = Strip Path(path=w2382) -> (stripped path=w2375:path, name=w2376:string)
                n1157 = Set File Position(refnum=w2378) -> (refnum out=w2377:refnum<file>)  [unwired: 3 in, 1 out]
                n1158 = local read "Data Output"() -> (w2391:T12)
                n1159 = call <vilib>:"Read File+ (string).vi"("count"=w2393, "refnum"=w2377) -> ("string"=w2394:string, "dup refnum"=w2395:refnum<file>)  [unwired: 5 in, 3 out]
                n1160 = Unflatten From String(type=w2393, binary string=w2394) -> (value=w2392:i32)  [unwired: 3 in, 2 out]
                n1161 = Bundle("Data Output"=w2391, "output cluster"=T26 {"Impulse Positions"=[], "Old Impulse positions for Undo"=[], "No. Imp"=0}) -> (w2390:T51)  [unwired: 1 in]
                n1162 = call <vilib>:"Read File+ (string).vi"("count"=w2392, "refnum"=w2395) -> ("string"=w2396:string, "dup refnum"=w2374:refnum<file>)  [unwired: 5 in, 3 out]
                n1163 = Close File(refnum=w2374) -> ()  [unwired: 1 in, 2 out]
                n1164 = Unflatten From String(type=w2390, binary string=w2396) -> (value=w2389:T51)  [unwired: 3 in, 2 out]
                n1165 = Unbundle(w2389) -> ("Data Output"=w2381:T12, "output cluster"=w2385:T26)
                n1166 = Unbundle By Name(w2385) -> ("Impulse Positions"=w2384:T11, "No. Imp"=w2383:i32)
                n1167 = Bundle By Name(cluster=w2386, "filename"=w2376, "Experiment data path"=w2375, "Experiment Parameters 2"=T24 {"Subject"="", "Strain"="", "Rotation plane"="", "Experimenter"="", "Trial"=0.0, "Time"=0.0}, "Experiment Parameters"=T25 {"Freq"=0.0, "Vel"=0, "Acc"=0, "Stimulus"=""}, "Data File"=w2381, "Impulse Positions"=w2384, "No. Imp"=w2383) -> (w2388:T30)
              }
              frame "CANCEL" {
              }
            }
          }
          frame Enabled {
            n1168 = case shown="False" w2401 {
              tunnel: w2400 -> [w2405 _]
              tunnel: w2399 -> [w2404 w2406]
              tunnel: [w2403 w2406] -> w2398
              frame False {
                # "Dialog not cancelled. Load the specified file."
                n1169 = call "Load LVS.vi"("LVS Data (in)"=w2404, "Path (in)"=w2405) -> ("error out"=w2402:errorcluster, "LVS Data (out)"=w2403:T30)  [unwired: 7 in, 1 out]
                n1170 = call <vilib>:"Simple Error Handler.vi"("error in (no error)"=w2402) -> ()  [unwired: 4 in, 5 out]
              }
              frame True {
                # "Dialog cancelled. Do nothing."
              }
            }
          }
        }
        n1171 = Bundle By Name(cluster=w2309, "DC file"=path "") -> (w2308:T17)
      }
      frame "Append Data" {
        w2443 = 4 ("count")
        n1172 = File Dialog(6:"*.lvs" ("pattern"), 7:"Select Data File:" ("prompt")) -> (0:w2423:errorcluster, 3:w2439:path)  [unwired: 5 in, 2 out]
        n1173 = Unbundle(w2423) -> ()  [unwired: 3 out]
        n1174 = call <vilib>:"Open_Create_Replace File.vi"("file path"=w2439) -> ("refnum"=w2446:refnum<file>)  [unwired: 7 in, 3 out]
        n1175 = local read "Data Output"() -> (w2421:T12)
        n1176 = call <vilib>:"Read File+ (string).vi"("count"=w2443, "refnum"=w2446) -> ("string"=w2444:string, "dup refnum"=w2445:refnum<file>)  [unwired: 5 in, 3 out]
        n1177 = Unflatten From String(type=w2443, binary string=w2444) -> (value=w2442:i32)  [unwired: 3 in, 2 out]
        n1178 = call <vilib>:"Read File+ (string).vi"("count"=w2442, "refnum"=w2445) -> ("string"=w2447:string)  [unwired: 5 in, 4 out]
        n1179 = Bundle("Data Output"=w2421, "Data OUT"=w2420) -> (w2422:T39)  [unwired: 1 in]
        n1180 = Unflatten From String(type=w2422, binary string=w2447) -> (value=w2419:T39)  [unwired: 3 in, 2 out]
        n1181 = Unbundle By Name(w2420) -> ("Impulse Positions"=w2429:T11)
        n1182 = Unbundle(w2419) -> ("Data Output"=w2418:T12, "Data OUT"=w2417:T30)
        n1183 = Unbundle By Name(w2417) -> ("Impulse Positions"=w2432:T11)
        n1184 = Unbundle By Name(w2421) -> ("Data Channels"=w2435:dbl[][])
        n1185 = Unbundle By Name(w2418) -> ("Data Channels"=w2437:dbl[][])
        n1186 = Transpose 2D Array(2D array=w2435) -> (transposed array=w2426:dbl[][])
        n1187 = Transpose 2D Array(2D array=w2437) -> (transposed array=w2425:dbl[][])
        n1188 = Build Array (concatenate)(w2426, w2425) -> (w2436:dbl[][])
        n1189 = Array Size(array=w2426) -> (size(s)=w2434:i32[])
        n1190 = Index Array(array=w2434, index=0) -> (element=w2431:i32)
        n1191 = for {
          tunnel: w2432 -> [w2455] mode=indexing
          tunnel: w2431 -> [w2450]
          tunnel: [w2449] -> w2430 mode=indexing
          n1192 = Unbundle By Name(w2455) -> ("Start"=w2454:i32, "End"=w2453:i32)
          n1193 = Add(x=w2450, y=w2454) -> (x+y=w2451:i32)
          n1194 = Add(x=w2453, y=w2450) -> (x+y=w2452:i32)
          n1195 = Bundle By Name(cluster=w2455, "Start"=w2451, "End"=w2452) -> (w2449:T18)
        }
        n1196 = Transpose 2D Array(2D array=w2436) -> (transposed array=w2424:dbl[][])
        n1197 = Bundle By Name(cluster=w2421, "Data Channels"=w2424) -> (w2428:T12)
        n1198 = Build Array (concatenate)(w2429, w2430) -> (w2427:T11)
        n1199 = local write "Impulse Positions"(w2427) -> ()
        n1200 = local write "Data Output"(w2428) -> ()
        n1201 = Bundle By Name(cluster=w2420, "Impulse Positions"=w2427) -> (w2438:T30)
      }
      frame "Horizontal Align" {
        n1202 = local read "Data Output"() -> (w2463:T12)
        n1203 = Unbundle By Name(w2458) -> ("Impulse Positions"=w2459:T11)
        n1204 = Unbundle By Name(w2463) -> ("Channel List"=w2462:string[])
        n1205 = local read "Impulse Plane 2"() -> (w2470:T9)
        n1206 = local read "Impulse dir"() -> (w2472:bool)
        n1207 = Index Array(array=w2462, index="Aligning Channel") -> (element=w2464:string)
        n1208 = property on="Impulse Trace" class="WFGraph (strict)"() -> ("Cursor.Cursor Position:Cursor X"=w2469:dbl, "Cursor.Cursor Position:Cursor Y"=w2468:dbl)  [unwired: 2 in, 2 out]
        n1209 = call "Align Impulses.vi"("Data Input"=w2463, "Impulse Direction +ve?"=w2472, "Alignment"=enum16{"Vertically", "Horizontally"}."Horizontally", "Display"=w2464, "Impulse Plane"=w2470, "Impulse Positions (in)"=w2459, "X Level"=w2469, "Y Level"=w2468) -> ("Impulse Positions (out)"=w2466:T11)  [unwired: 11 in]
        n1210 = local write "Impulse Positions"(w2466) -> ()
        n1211 = call "Add History.vi"("Data IN"=w2458, "Impulse Positions"=w2459) -> ("Data OUT"=w2457:T30)  [unwired: 9 in]
        n1212 = Bundle By Name(cluster=w2457, "Impulse Positions"=w2466) -> (w2467:T30)
      }
      frame "Vertical Align" {
        n1213 = local read "Data Output"() -> (w2480:T12)
        n1214 = Unbundle By Name(w2476) -> ("Impulse Positions"=w2477:T11)
        n1215 = local read "Aligning Channel"() -> (w2483:u16)
        n1216 = Unbundle By Name(w2480) -> ("Channel List"=w2481:string[])
        n1217 = local read "Impulse Plane 2"() -> (w2488:T9)
        n1218 = local read "Impulse dir"() -> (w2490:bool)
        n1219 = Index Array(array=w2481, index=w2483) -> (element=w2482:string)
        n1220 = property on="Impulse Trace" class="WFGraph (strict)"() -> ("Cursor.Cursor Position:Cursor X"=w2487:dbl, "Cursor.Cursor Position:Cursor Y"=w2486:dbl)  [unwired: 2 in, 2 out]
        n1221 = call "Align Impulses.vi"("Data Input"=w2480, "Impulse Direction +ve?"=w2490, "Alignment"=enum16{"Vertically", "Horizontally"}."Vertically", "Display"=w2482, "Impulse Plane"=w2488, "Impulse Positions (in)"=w2477, "X Level"=w2487, "Y Level"=w2486) -> ("Impulse Positions (out)"=w2484:T11)  [unwired: 11 in]
        n1222 = local write "Impulse Positions"(w2484) -> ()
        n1223 = call "Add History.vi"("Data IN"=w2476, "Impulse Positions"=w2477) -> ("Data OUT"=w2475:T30)  [unwired: 9 in]
        n1224 = Bundle By Name(cluster=w2475, "Impulse Positions"=w2484) -> (w2485:T30)
      }
      frame "Delete Impulse" {
        # "Trace to delete if Esc or Delete was pressed."
        # "Traces to delete if paint delete was used."
        # "Impulses must be deleted in descending order so that their plot number continues to make sense during deletion."
        n1225 = Unbundle By Name(w2508) -> ("Delete-Array"=w2494:i32[])
        n1226 = local read "Trace"() -> (w2499:i32)
        n1227 = Unbundle By Name(w2506) -> ("Impulse Positions"=w2507:T11, "No. Imp"=w2492:i32)
        n1228 = Build Array(w2499) -> (w2496:i32[])
        n1229 = Array Size(array=w2494) -> (size(s)=w2498:i32)
        n1230 = Greater Than 0?(x=w2498) -> (x > 0?=w2497:bool)
        n1231 = Quotient & Remainder(x=w2494, y=w2492) -> (x-y*floor(x/y)=w2493:i32[])  [unwired: 1 out]
        n1232 = Select(t=w2493, s=w2497, f=w2496) -> (s? t:f=w2495:i32[])
        n1233 = local read "Impulse Plane 2"() -> (w2511:T9)
        n1234 = local read "Impulse dir"() -> (w2512:bool)
        n1235 = call-poly <userlib>:"Sort Array__ogtk.vi"("Order"=enum16{"ascending", "descending"}."descending", "Array in"=w2495) -> ("Sorted Array out"=w2501:i32[])  [unwired: 8 in, 1 out]
        n1236 = for {
          tunnel: w2512 -> [w2527]
